vi "ConfigStdWF.vi"(0 "object in":refnum<class "AFG3022B.lvclass">, 2 "Configdatastd":T1, 5 "error in (no error)":errorcluster) -> (14 "object out":refnum<class "AFG3022B.lvclass">, 19 "error out":errorcluster)   [LabVIEW 2019, in "AFG3022B.lvclass"]
uses:
  AFG3022B.lvclass
  AFG3022B.lvclass/AFG3022B.ctl
  Tektronix AFG 3000 Series/Tektronix AFG 3000 Series.lvlib
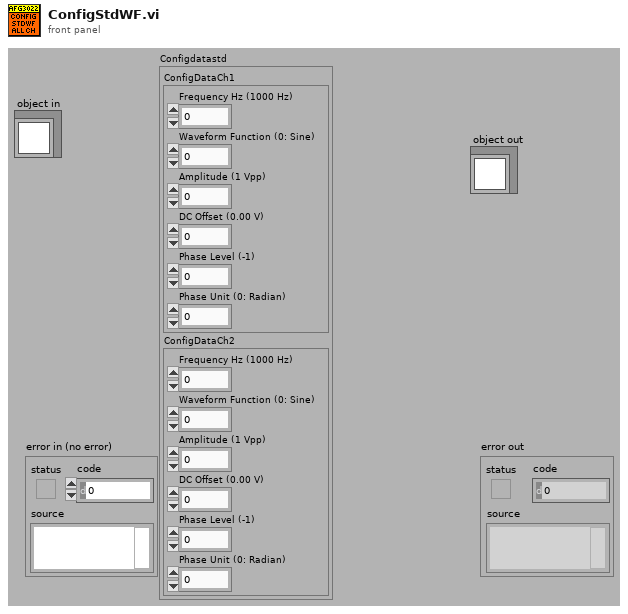
[diagram p1: front panel]
types:
  T1 = cluster{"ConfigDataCh1":cluster{"Frequency Hz (1000 Hz)":dbl, "Waveform Function (0: Sine)":u16, "Amplitude (1 Vpp)":dbl, "DC Offset (0.00 V)":dbl, "Phase Level (-1)":dbl, "Phase Unit (0: Radian)":u16}, "ConfigDataCh2":cluster{"Frequency Hz (1000 Hz)":dbl, "Waveform Function (0: Sine)":u16, "Amplitude (1 Vpp)":dbl, "DC Offset (0.00 V)":dbl, "Phase Level (-1)":dbl, "Phase Unit (0: Radian)":u16}}
  T2 = cluster{"Frequency Hz (1000 Hz)":dbl, "Waveform Function (0: Sine)":u16, "Amplitude (1 Vpp)":dbl, "DC Offset (0.00 V)":dbl, "Phase Level (-1)":dbl, "Phase Unit (0: Radian)":u16}
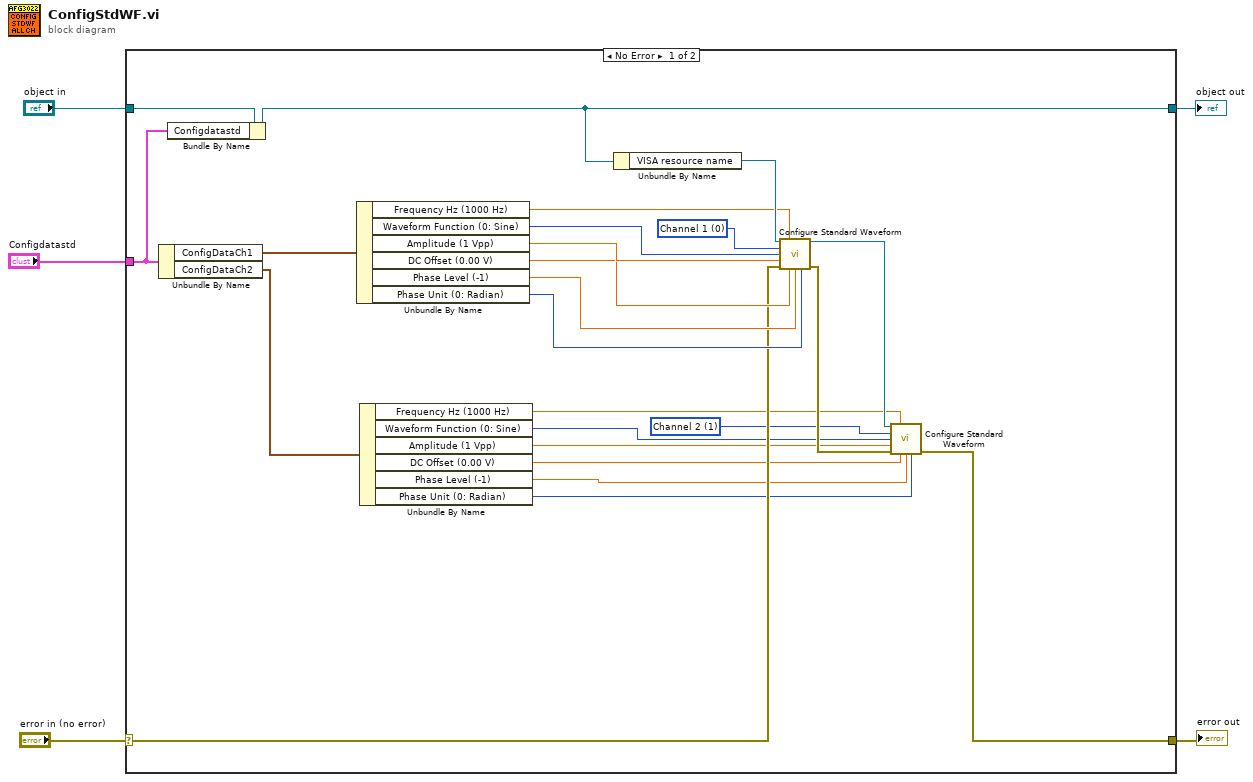
[diagram p0: block diagram]
diagram:
  n1 = case shown="No Error" "error in (no error)" {
    selector: "error in (no error)" -> [w20 w31]
    tunnel: [w18 w31] -> w4
    tunnel: [w21 w30] -> w2
    tunnel: "object in" -> [w29 w30]
    tunnel: "Configdatastd" -> [w15 _]
    frame No Error {
      w11 = u16 1 items=["Channel 1", "Channel 2"] ("Channel (0: Channel 1)")
      w17 = u16 0 items=["Channel 1", "Channel 2"] ("Channel (0: Channel 1)")
      n2 = Unbundle By Name(w15) -> ("ConfigDataCh1"=w14:T2, "ConfigDataCh2"=w13:T2)
      n3 = Bundle By Name(cluster=w29, "Configdatastd"=w15) -> (w21:refnum<class "AFG3022B.lvclass">)
      n4 = Unbundle By Name(w14) -> ("Frequency Hz (1000 Hz)"=w27:dbl, "Waveform Function (0: Sine)"=w26:u16, "Amplitude (1 Vpp)"=w25:dbl, "DC Offset (0.00 V)"=w24:dbl, "Phase Level (-1)"=w23:dbl, "Phase Unit (0: Radian)"=w22:u16)
      n5 = Unbundle By Name(w13) -> ("Frequency Hz (1000 Hz)"=w12:dbl, "Waveform Function (0: Sine)"=w10:u16, "Amplitude (1 Vpp)"=w9:dbl, "DC Offset (0.00 V)"=w8:dbl, "Phase Level (-1)"=w7:dbl, "Phase Unit (0: Radian)"=w6:u16)
      n6 = Unbundle By Name(w21) -> ("VISA resource name"=w28:refnum<visa-resource-name>)
      n7 = call "Configure Standard Waveform.vi"("VISA resource name"=w28, "Frequency (1000 Hz)"=w27, "Channel (0: Channel 1)"=w17, "Waveform Function (0: Sine)"=w26, "Amplitude (1 Vpp)"=w25, "error in (no error)"=w20, "DC Offset (0.00 V)"=w24, "Phase Level (-1)"=w23, "Phase Unit (0: Radian)"=w22) -> ("VISA resource name out"=w16:refnum<visa-resource-name>, "error out"=w19:errorcluster)  [unwired: 5 in]
      n8 = call "Configure Standard Waveform.vi"("VISA resource name"=w16, "Frequency (1000 Hz)"=w12, "Channel (0: Channel 1)"=w11, "Waveform Function (0: Sine)"=w10, "Amplitude (1 Vpp)"=w9, "error in (no error)"=w19, "DC Offset (0.00 V)"=w8, "Phase Level (-1)"=w7, "Phase Unit (0: Radian)"=w6) -> ("error out"=w18:errorcluster)  [unwired: 5 in, 1 out]
    }
    frame Error {
    }
  }
  "error out" <- w4
  "object out" <- w2
